vi "TimbreGenerator (3).vi"() -> ()   [LabVIEW 2022 SP3]
uses:
  <vilib>/express/express analysis/Spectral/Block/exnSpectralBlock spectral measurements RMS poly.vi
  <vilib>/express/express analysis/Spectral/Block/exnSpectralBlock spectral measurements RMS DDT.vi
  <vilib>/express/express analysis/Spectral/XNode/ExpressSpectralMeasurementsBlockNode.xnode
panel:
  in  "Tab Control 3":enum32{"Page 1"}(tab)
  in  "Play Simulated Waveform":bool
  in  "Record Sound":bool
  in  "Play Mic Input":bool
  in  "Duration (s)":dbl=5.0
  in  "Tab Control 2":T1(tab)
  in  "Frequencies":dbl[](array[slide])=[2653.061224489796, 2653.061224489796, 0.0, 0.0, 0.0, 0.0, 0.0, 0.0, 0.0] scale=0.0..20000.0
  in  "Phases":dbl[](array[slide])=[0.0, 0.0, 0.0, 0.0, 0.0, 0.0, 0.0, 0.0, 0.0] scale=0.0..360.0
  in  "Signal Types":i32[](array[knob])=[0, 0, 0, 0, 0, 0, 0, 0, 0] scale=0.0..3.0
  in  "Amplitudes":dbl[](array[slide])=[1.0, 1.0, 1.0, 1.0, 1.0, 1.0, 1.0, 1.0, 0.0] scale=0.0..1.0
  in  "Tab Control":T2(tab)
  out "Simulated Sound Waveform":dynamicdata(graph)=[{"t0"=timestamp(229.53729581832886 s since 1904-01-01), "dt"=2.2675736961451248e-05, "Y"=array[4410 elements], "attributes"=variant("NI_ChannelName"=variant(string "Sine"), "NI_ExpIsRelativeTime"=variant(bool TRUE), "NI_ExpStartTimeStamp"=variant(timestamp timestamp(3789516260.29932 s since 1904-01-01)), "NI_ExpTimeStamp"=variant(timestamp timestamp(3789516489.836616 s since 1904-01-01)), "NI_ExpXDimension"=variant(string "t"))}]
  out "Mic Input":dynamicdata(graph)=[{"t0"=timestamp(3789516378.597457 s since 1904-01-01), "dt"=2.2675736961451248e-05, "Y"=array[220500 elements]}] caption="Data"
  out "Mic Input FFT":dynamicdata(graph)=[{"t0"=timestamp(0 s since 1904-01-01), "dt"=0.2, "Y"=array[110250 elements], "attributes"=variant("NI_ChannelName"=variant(string "FFT - (RMS)"))}]
  out "Simulated FFT":dynamicdata(graph)=[{"t0"=timestamp(0 s since 1904-01-01), "dt"=10.0, "Y"=array[2205 elements], "attributes"=variant("NI_ChannelName"=variant(string "Sine (FFT - (RMS))"), "NI_ExpIsRelativeTime"=variant(bool TRUE), "NI_ExpStartTimeStamp"=variant(timestamp timestamp(3789516260.29932 s since 1904-01-01)), "NI_ExpTimeStamp"=variant(timestamp timestamp(3789516489.836616 s since 1904-01-01)), "NI_ExpXDimension"=variant(string "f"), "NI_OriginalChannelName"=variant(string "Sine"))}]
  out "Filter On":bool
  in  "Filter Toggle":bool
  in  "Cutoff Frequency (High End)":dbl=1600.0
  in  "Cutoff Frequency (Low End)":dbl=1500.0 min=0.0 max=22000.0 step=10.0
  in  "Filter Type":i32(knob)=2 scale=0.0..2.0
  in  "stop":bool
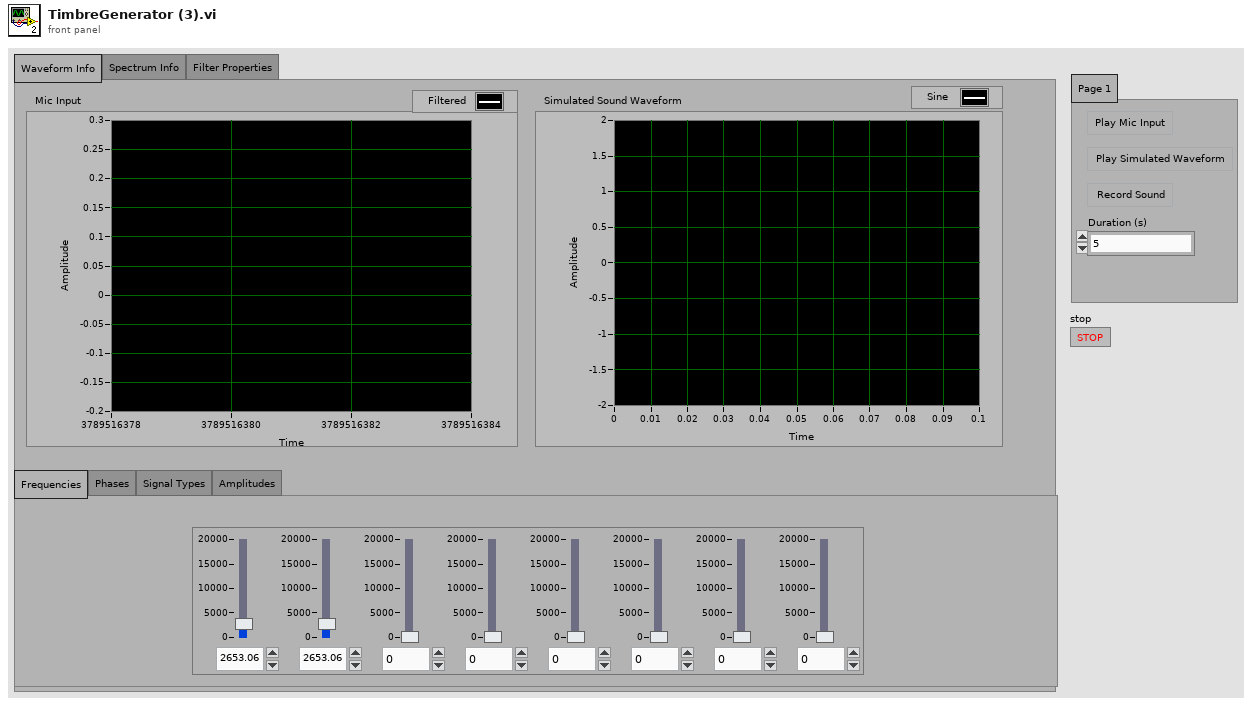
[diagram p1: front panel]
types:
  T1 = enum32{"Frequencies", "Phases", "Signal Types", "Amplitudes"}
  T2 = enum32{"Waveform Info", "Spectrum Info", "Filter Properties"}
  T3 = cluster{"averaging mode":u16, "weighting mode":u16, "number of averages":u32}
  T4 = cluster{"dB On (F)":bool, "unwrap phase (F)":bool, "convert to degree (F)":bool}
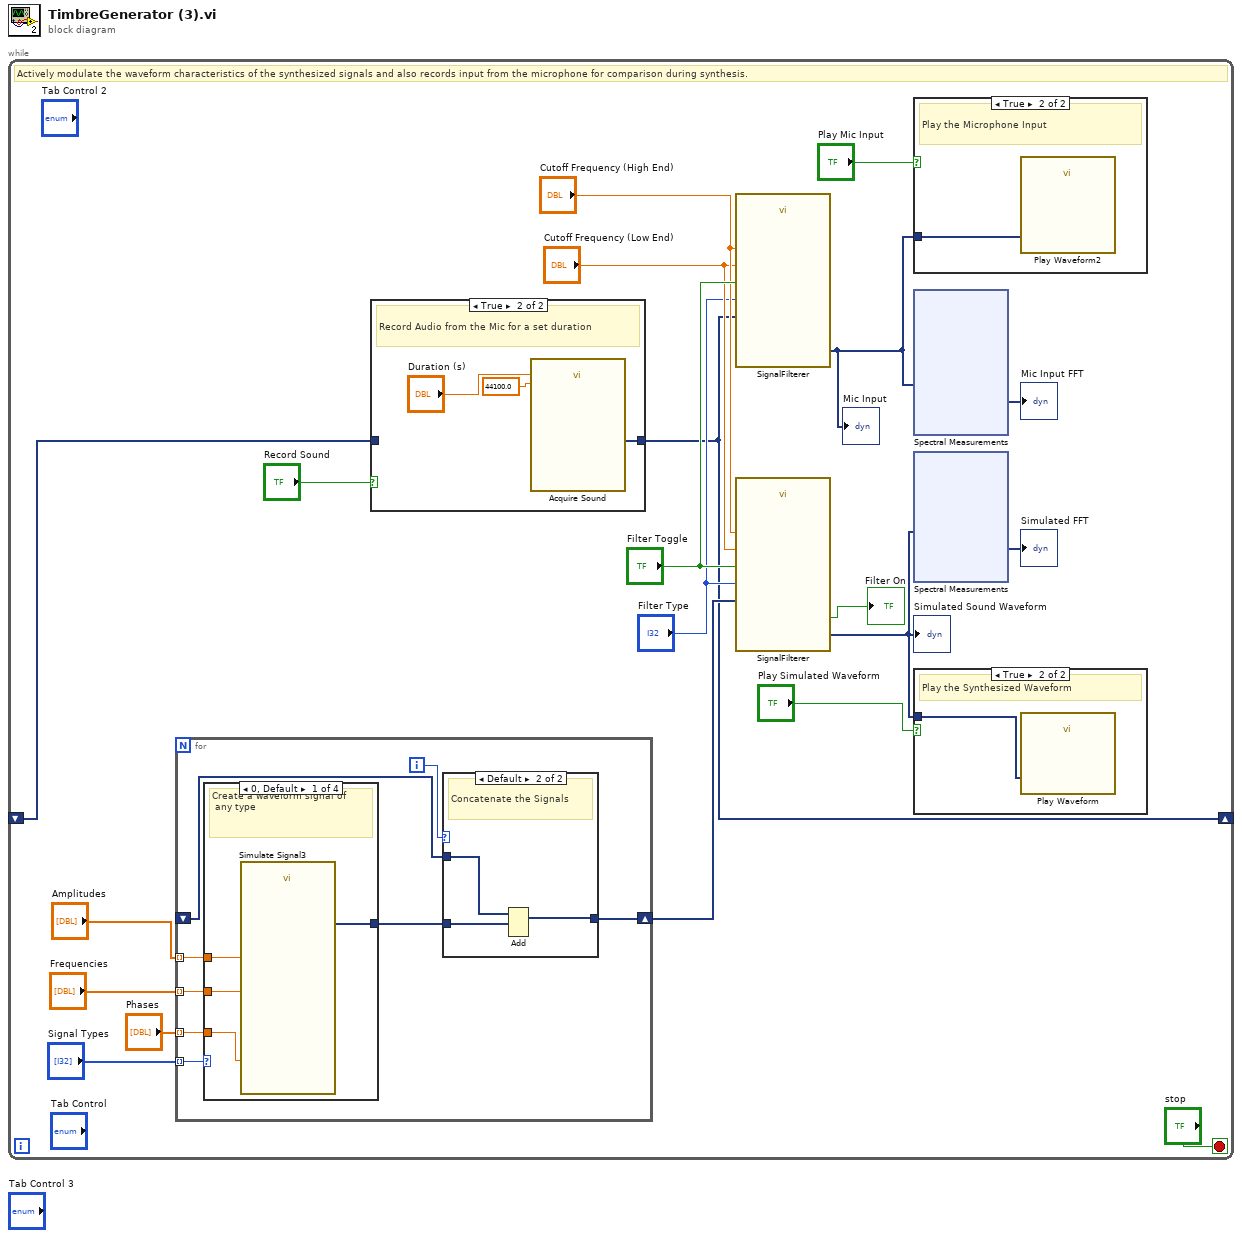
[diagram p0: block diagram]
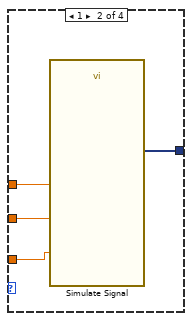
[diagram p5: hidden frame]
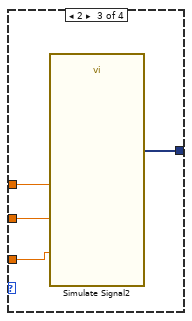
[diagram p6: hidden frame]
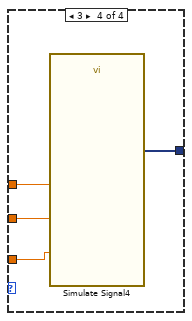
[diagram p7: hidden frame]
diagram:
  n1 = while {
    shift-right: [w6] -> _
    shift-left: _ -> [w5]
    stop <- "stop" stop-if-true
    # "Actively modulate the waveform characteristics of the synthesized signals and also records input from the microphone for comparison during synthesis."
    n2 = for {
      tunnel: "Frequencies" -> [w44] mode=indexing
      shift-right: [w39] -> w14
      shift-left: _ -> [w40]
      tunnel: "Phases" -> [w43] mode=indexing
      tunnel: "Signal Types" -> [w38] mode=indexing
      tunnel: "Amplitudes" -> [w37] mode=indexing
      i -> [w42]
      n3 = case shown="0, Default" w38 {
        tunnel: w44 -> [w47 w52 w56 w59]
        tunnel: w43 -> [w46 w51 w55 w58]
        tunnel: [w48 w50 w54 w60] -> w41
        tunnel: w37 -> [w45 w49 w53 w57]
        frame 0, Default {
          # "Create a waveform signal of\n any type"
          n4 = call "Simulate Signal3"("Frequency"=w47, "Amplitude"=w45, "Phase"=w46) -> ("Sine"=w48:dynamicdata)  [unwired: 11 in, 1 out]
        }
        frame 1 {
          n5 = call "Simulate Signal"("Frequency"=w52, "Amplitude"=w49, "Phase"=w51) -> ("Square"=w50:dynamicdata)  [unwired: 11 in, 1 out]
        }
        frame 2 {
          n6 = call "Simulate Signal2"("Frequency"=w56, "Amplitude"=w53, "Phase"=w55) -> ("Triangle"=w54:dynamicdata)  [unwired: 11 in, 1 out]
        }
        frame 3 {
          n7 = call "Simulate Signal4"("Frequency"=w59, "Amplitude"=w57, "Phase"=w58) -> ("Sawtooth"=w60:dynamicdata)  [unwired: 11 in, 1 out]
        }
      }
      n8 = case shown="Default" w42 {
        tunnel: w41 -> [w61 w64]
        tunnel: w40 -> [_ w63]
        tunnel: [w61 w62] -> w39
        frame 0 {
        }
        frame Default {
          # "Concatenate the Signals"
          n9 = Add(1:w64, 2:w63) -> (0:w62:dynamicdata)  [unwired: 1 in, 1 out]
        }
      }
    }
    n10 = case shown="True" "Record Sound" {
      tunnel: [w32 w33] -> w6
      tunnel: w5 -> [w32 _]
      frame False {
      }
      frame True {
        # "Record Audio from the Mic for a set duration"
        n11 = call "Acquire Sound"("Duration (s)"="Duration (s)", "Sample rate (Hz)"=44100.0) -> ("Data"=w33:dynamicdata)  [unwired: 16 in, 1 out]
      }
    }
    n12 = call "SignalFilterer.vi"("Cutoff Frequency (Low End)"="Cutoff Frequency (Low End)", "Cutoff Frequency (High End)"="Cutoff Frequency (High End)", "Sawtooth"=w6, "Filter Type"="Filter Type", "Filter Toggle"="Filter Toggle") -> ("Filtered Signal"=w1:dynamicdata)  [unwired: 5 in, 1 out]
    "Mic Input" <- w1
    n13 = call "SignalFilterer.vi"("Cutoff Frequency (Low End)"="Cutoff Frequency (Low End)", "Cutoff Frequency (High End)"="Cutoff Frequency (High End)", "Sawtooth"=w14, "Filter Type"="Filter Type", "Filter Toggle"="Filter Toggle") -> ("Filtered Signal"=w12:dynamicdata, "Filter On"=→"Filter On":bool)  [unwired: 5 in]
    "Simulated Sound Waveform" <- w12
    n14 = case shown="True" "Play Mic Input" {
      tunnel: w1 -> [_ w21]
      frame False {
      }
      frame True {
        # "Play the Microphone Input"
        n15 = call "Play Waveform2"("Data"=w21) -> ()  [unwired: 18 in, 1 out]
      }
    }
    n16 = xnode "Spectral Measurements"("Signals"=w1) -> ("FFT - (RMS)"=→"Mic Input FFT":dynamicdata)  [unwired: 1 in, 2 out]
    n17 = xnode "Spectral Measurements"("Signals"=w12) -> ("FFT - (RMS)"=→"Simulated FFT":dynamicdata)  [unwired: 1 in, 2 out]
    n18 = case shown="True" "Play Simulated Waveform" {
      tunnel: w12 -> [_ w36]
      frame False {
      }
      frame True {
        # "Play the Synthesized Waveform"
        n19 = call "Play Waveform"("Data"=w36) -> ()  [unwired: 18 in, 1 out]
      }
    }
  }
